vi "Temp Value Changed.vi"(8 "error in (no error)":errorcluster, 10 "Current Temp. Value":dbl, 11 "Heating Control Interface in":refnum<class "Heating Control Interface.lvclass">) -> (0 "error out":errorcluster, 3 "Heating Control Interface out":refnum<class "Heating Control Interface.lvclass">)   [LabVIEW 2021, in "Logic.lvlib" / "Heating Control Interface.lvclass"]
uses:
  Heating Control Interface.lvclass
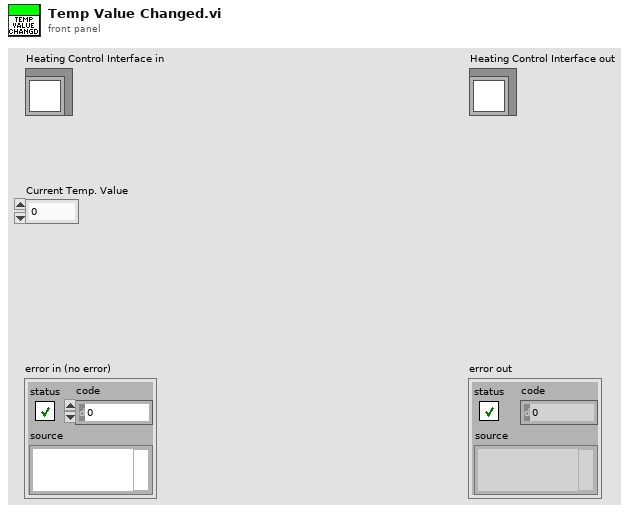
[diagram p1: front panel]
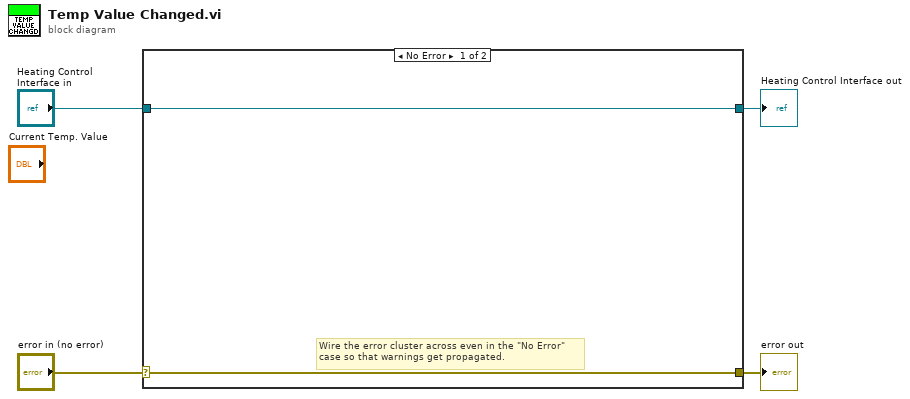
[diagram p0: block diagram]
diagram:
  n1 = case shown="No Error" "error in (no error)" {
    selector: "error in (no error)" -> [w5 w8]
    tunnel: [w5 w8] -> w3
    tunnel: [w6 w7] -> w1
    tunnel: "Heating Control Interface in" -> [w6 w7]
    frame No Error {
      # "Wire the error cluster across even in the \"No Error\"\ncase so that warnings get propagated."
    }
    frame Error {
    }
  }
  "error out" <- w3
  "Heating Control Interface out" <- w1
